vi "Read U8.vi"(8 "error in (no error)":errorcluster, 10 "Tag":string, 11 "Var Bus in":refnum<class "Var Bus.lvclass">) -> (0 "error out":errorcluster, 2 "Numeric":u8, 3 "Var Bus out":refnum<class "Var Bus.lvclass">)   [LabVIEW 2021, in "Var Bus.lvclass"]
uses:
  Var Bus.lvclass
  Var Bus.lvclass/Var Bus.ctl
  LV_Abstract/Source/Abs_Types/Numeric/Abs_Numeric.lvclass
  Var Index/Var_Index.lvclass
  C:/Users/Tim/Documents/LabVIEW/2021/Data Classes/Source/Abs_Types/Value/Abs_Value.lvclass
  C:/Users/Tim/Documents/LabVIEW/2021/Data Classes/Source/Abs_Types/Type/Abs_Type.lvclass
  C:/Users/Tim/Documents/LabVIEW/2021/Var Bus/Source/Var Index/Var_Index.lvclass
  LV_Abstract/Source/Abs_Types/Value/Abs_Value.lvclass
  C:/Users/Tim/Documents/LabVIEW/2021/Data Classes/Source/Abs_Types/Numeric/Abs_Numeric.lvclass
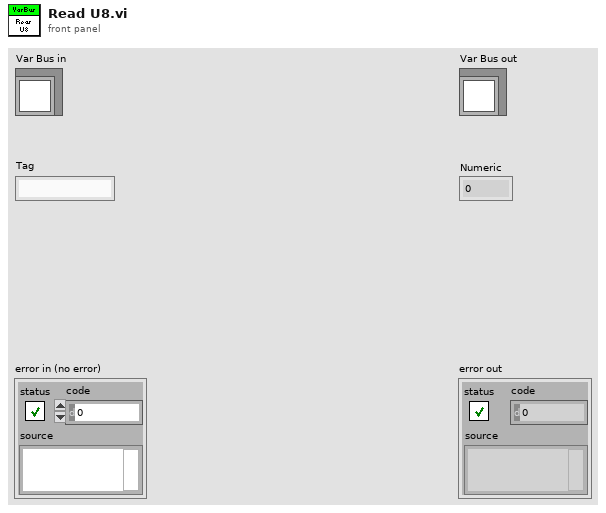
[diagram p1: front panel]
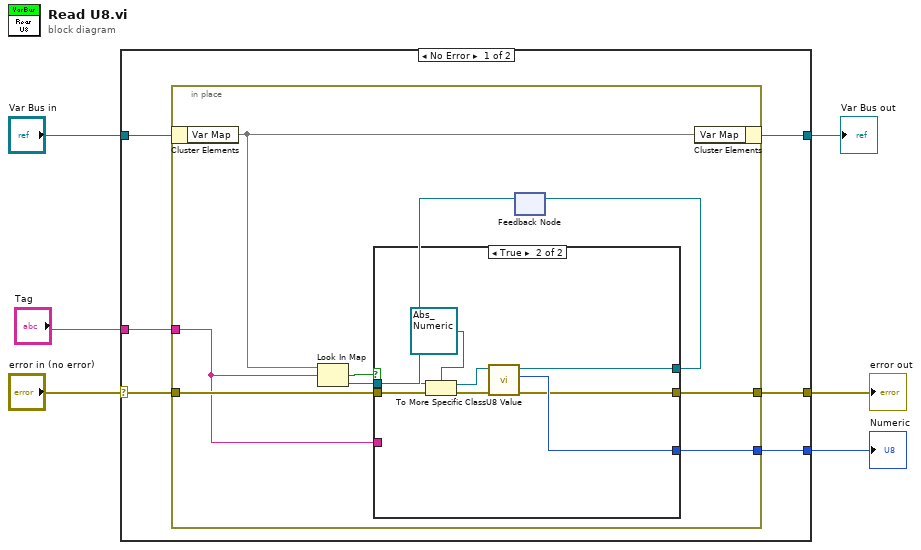
[diagram p0: block diagram]
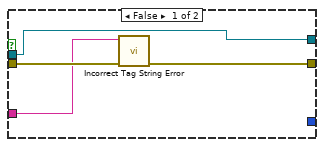
[diagram p2: hidden frame]
diagram:
  n1 = case shown="No Error" "error in (no error)" {
    selector: "error in (no error)" -> [w10 w35]
    tunnel: [w8 w35] -> w5
    tunnel: [w9 w34] -> w3
    tunnel: "Var Bus in" -> [w12 w34]
    tunnel: "Tag" -> [w11 _]
    tunnel: [w7 _] -> w1
    frame No Error {
      n2 = in-place {
        in-place-border: w11 -> [w14]
        in-place-border: w10 -> [w20]
        in-place-border: [w17] -> w8
        in-place-border: [w16] -> w7
        n3 = in-place-cluster #1(w12) -> ("Var Map"=w21:map{string, refnum<class "Var_Index.lvclass">})
        n4 = feedback #2() -> (w18:refnum<class "Abs_Value.lvclass">)  [unwired: 1 in]
        n5 = Look In Map(map=w21, key=w14, default value=w18) -> (key not found?=w15:bool, value=w19:refnum<class "Var_Index.lvclass">)
        n6 = case shown="True" w15 {
          tunnel: w20 -> [w25 w33]
          tunnel: [w24 w28] -> w17
          tunnel: [_ w29] -> w16
          tunnel: w14 -> [w23 _]
          tunnel: w19 -> [w22 w27]
          tunnel: [w22 w26] -> w13
          frame False {
            n7 = call "Incorrect Tag String Error.vi"("error in (no error)"=w25, "Tag"=w23) -> ("error out"=w24:errorcluster)  [unwired: 9 in]
          }
          frame True {
            n8 = To More Specific Class(target class=refnum<class "Abs_Numeric.lvclass"> refnum ("Abs_Numeric.lvclass"), reference=w27, error in=w33) -> (specific class reference=w30:refnum<class "Abs_Numeric.lvclass">, error out=w31:errorcluster)
            n9 = call-dynamic "U8 Value.vi"("error in (no error)"=w31, "Numeric in"=w30) -> ("error out"=w28:errorcluster, "U8"=w29:u8, "Numeric out"=w26:refnum<class "Abs_Numeric.lvclass">)  [unwired: 7 in]
          }
        }
        n10 = feedback-in #2(w13) -> ()
        n11 = in-place-cluster #1("Var Map"=w21) -> (w9:refnum<class "Var Bus.lvclass">)
      }
    }
    frame Error {
    }
  }
  "error out" <- w5
  "Var Bus out" <- w3
  "Numeric" <- w1
